vi "Send Part based Initialization_DL.vi"(7 "Message Priority (Normal)":T2=enum."Normal", 8 "error in (no error)":errorcluster, 10 "Part Info":T1, 11 "Message Enqueuer":refnum<class "Message Enqueuer.lvclass">) -> (0 "error out":errorcluster, 3 "Message Enqueuer out":refnum<class "Message Enqueuer.lvclass">)   [LabVIEW 2019, in "Part based Initialization_DL Msg.lvclass"]
doc: "This VI sends the message to an actor."
uses:
  Part based Initialization_DL Msg.lvclass
  <vilib>/ActorFramework/Message Enqueuer/Message Enqueuer.lvclass
  C:/Program Files/National Instruments/LabVIEW 2019/vi.lib/ActorFramework/Message/Message.lvclass
  <vilib>/ActorFramework/Message Enqueuer/Message Priority.ctl
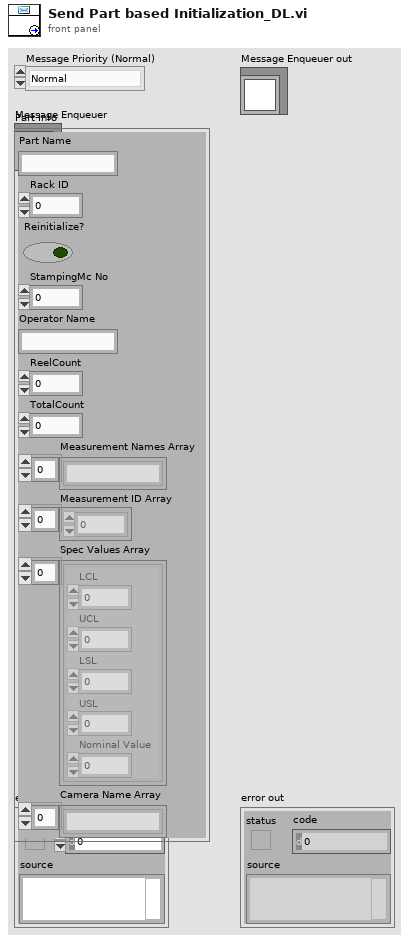
[diagram p1: front panel]
types:
  T1 = cluster{"Part Name":string, "Rack ID":u8, "Reinitialize?":bool, "StampingMc No":u64, "Operator Name":string, "ReelCount":u64, "TotalCount":u64, "Measurement Names Array":string[], "Measurement ID Array":u16[], "Spec Values Array":cluster{"LCL":dbl, "UCL":dbl, "LSL":dbl, "USL":dbl, "Nominal Value":dbl}[], "Camera Name Array":string[]}
  T2 = typedef "Actor Framework.lvlib/Message Enqueuer.lvclass/Message Priority.ctl" = enum16{"Low", "Normal", "High"}
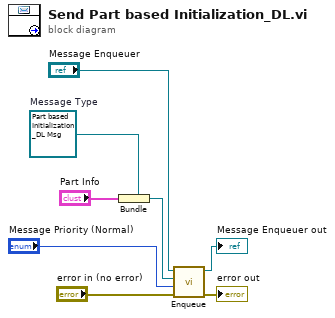
[diagram p0: block diagram]
diagram:
  w5 = refnum<class "Part based Initialization_DL Msg.lvclass"> refnum  # Message Type
  n1 = Bundle(cluster=w5, "Part Info") -> (w4:refnum<class "Part based Initialization_DL Msg.lvclass">)
  n2 = call <vilib>:"Enqueue.vi"("error in (no error)"="error in (no error)", "Message Priority (Normal)"="Message Priority (Normal)", "Message"=w4, "Message Enqueuer in"="Message Enqueuer") -> ("error out"=→"error out":errorcluster, "Message Enqueuer out"=→"Message Enqueuer out":refnum<class "Message Enqueuer.lvclass">)  [unwired: 6 in]
